vi "Horst.vi"() -> ()   [LabVIEW 2017]
uses:
  <vilib>/rvi/interface/nirviMethod/nirviMethod.xnode
  E:/HAGAR-V_ECD/FPGA-Programm_ECD.vi
  <vilib>/FPGAPlugInAG/cRIO-9035/niLvFpga_ReadFifo_cRIO-9035.vi
  <vilib>/rvi/errors/niLvFpgaMergeErrorWithErrorCode.vi
  FPGA Bitfiles/HAGAR-VECD_FPGATarget_FPGA-ProgrammECD_J-wKM9Jb3G8.lvbitx
panel:
  in  "Reglernummer":i32
  in  "Schleifenperiode":u32 caption="Anzahl (ms)"
  in  "Stopp":bool
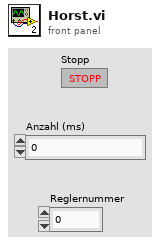
[diagram p1: front panel]
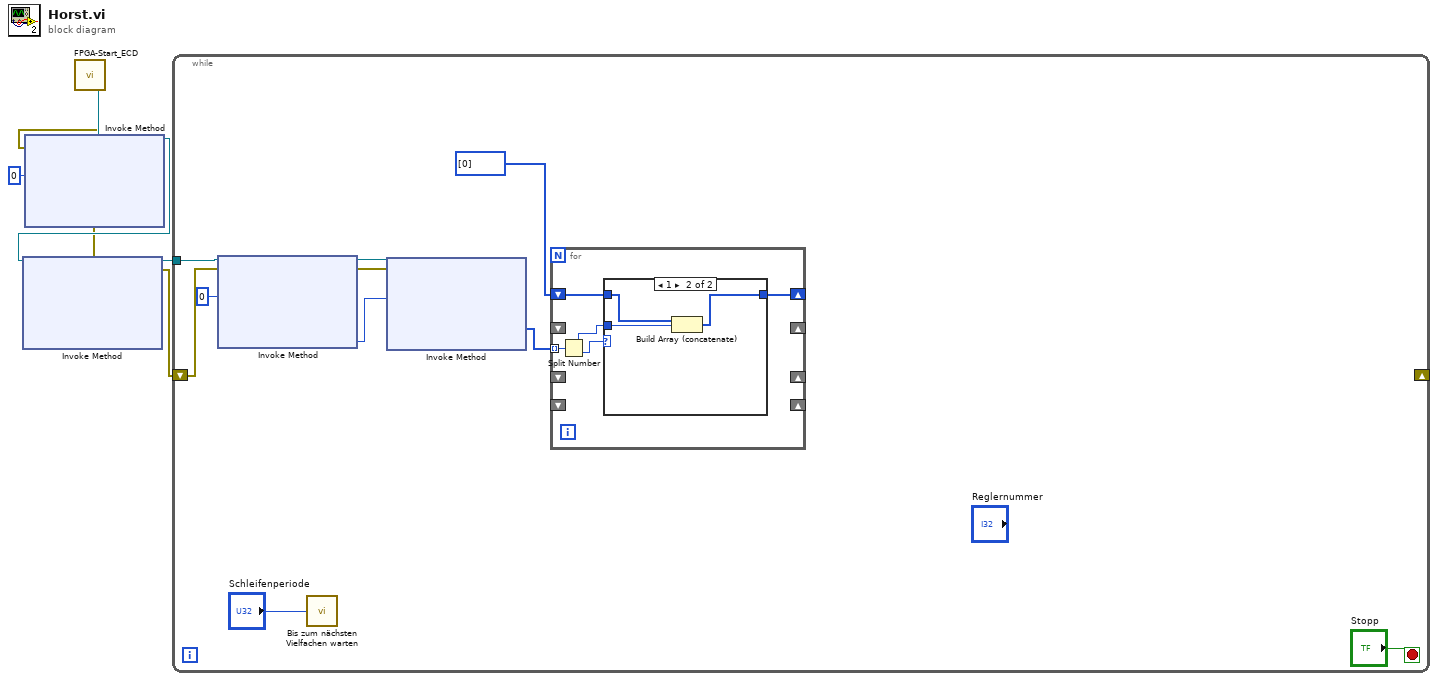
[diagram p0: block diagram]
diagram:
  n1 = call "FPGA-Start_ECD.vi"() -> ("error out"=w7:errorcluster, "FPGA-VI-Referenz (Ausgang)"=w8:refnum<k20>)  [unwired: 2 in]
  n2 = xnode "Invoke Method"("FPGA-VI-Referenz (Eingang)"=w8, "Fehler (Eingang)"=w7, "Anzahl der Elemente"=u32 0) -> ("FPGA-VI-Referenz (Ausgang)"=w5:refnum<k20>, "Fehler (Ausgang)"=w4:errorcluster, "Verbleibende Elemente"=w3:u32)  [unwired: 1 in, 1 out]
  n3 = xnode "Invoke Method"("FPGA-VI-Referenz (Eingang)"=w5, "Fehler (Eingang)"=w4, "Anzahl der Elemente"=w3) -> ("FPGA-VI-Referenz (Ausgang)"=w2:refnum<k20>, "Fehler (Ausgang)"=w1:errorcluster)  [unwired: 1 in, 2 out]
  n4 = while {
    shift-right: _ -> [_]
    shift-left: w1 -> [w14]
    tunnel: w2 -> [w16]
    stop <- "Stopp" stop-if-true
    n5 = xnode "Invoke Method"("FPGA-VI-Referenz (Eingang)"=w16, "Fehler (Eingang)"=w14, "Anzahl der Elemente"=u32 0) -> ("FPGA-VI-Referenz (Ausgang)"=w15:refnum<k20>, "Fehler (Ausgang)"=w13:errorcluster, "Verbleibende Elemente"=w11:u32)  [unwired: 1 in, 1 out]
    n6 = call "Bis zum nächsten Vielfachen warten"("Count(mSec)"="Schleifenperiode") -> ()  [unwired: 1 out]
    n7 = xnode "Invoke Method"("FPGA-VI-Referenz (Eingang)"=w15, "Fehler (Eingang)"=w13, "Anzahl der Elemente"=w11) -> ("Daten"=w10:u16[])  [unwired: 1 in, 3 out]
    n8 = for {
      tunnel: w10 -> [w23] mode=indexing
      shift-right: [w19] -> _
      shift-left: u8[] [0] -> [w20]
      shift-right: _ -> [_]
      shift-left: _ -> [_]
      shift-right: _ -> [_]
      shift-left: _ -> [_]
      shift-right: _ -> [_]
      shift-left: _ -> [_]
      n9 = Split Number(x=w23) -> (hi(x)=w21:u8, lo(x)=w22:u8)
      n10 = case shown="1" w22 {
        tunnel: w21 -> [_ w26]
        tunnel: w20 -> [w24 w27]
        tunnel: [w24 w25] -> w19
        frame 0, Default {
        }
        frame 1 {
          n11 = Build Array (concatenate)(w27, w26) -> (w25:u8[])
        }
      }
    }
  }
